vi "RSZVB Set Converter Source Frequency.vi"(4 "Numerator":i32, 5 "Sweep Type (0)":i32(ring) items=["Sweep", "CW/Fixed"], 6 "Offset":dbl format="%^.3e", 7 "Denominator":i32, 8 "error in (no error)":errorcluster {"code" format="%.0x"}, 9 "Port (1)":i32=1, 10 "Channel (1)":i32=1, 11 "VISA session":refnum<visa-resource-name>) -> (0 "error out":errorcluster {"code" format="%.0x"}, 3 "dup VISA session":refnum<visa-resource-name>)   [LabVIEW 2011]
doc: "Defines the converter source frequency at the converter port <Pt>.\n\nNotes:\n\n(1) This command is available for frequency converters with electronic attenuators R&S ZVA-ZxxxE.\n\nRemote-control command(s):\nSOURce<Ch>:FREQuency<Pt>:CONVersion:ARBitrary:CFRequency <numerator>, <denominator>, <offset>, CW | FIXed | SWEep"
uses:
  _utility/RSZVB Global Data.vi
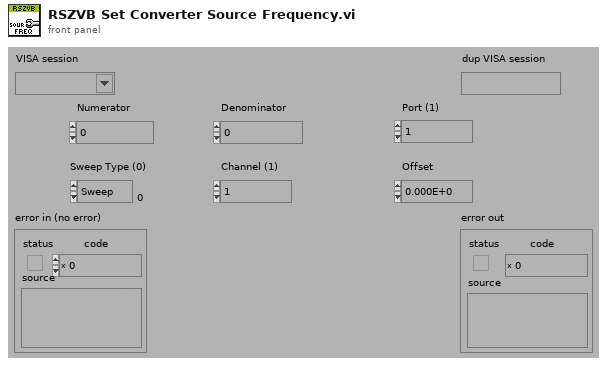
[diagram p1: front panel]
types:
  T1 = cluster{"Error Checking (T: On)":bool, "Installed Options":string[], "Data Valid?":bool, "Ports":i32, "Model":string[], "Option Checking (T: On)":bool}[]
  T2 = cluster{"Error Checking (T: On)":bool, "Installed Options":string[], "Data Valid?":bool, "Ports":i32, "Model":string[], "Option Checking (T: On)":bool}
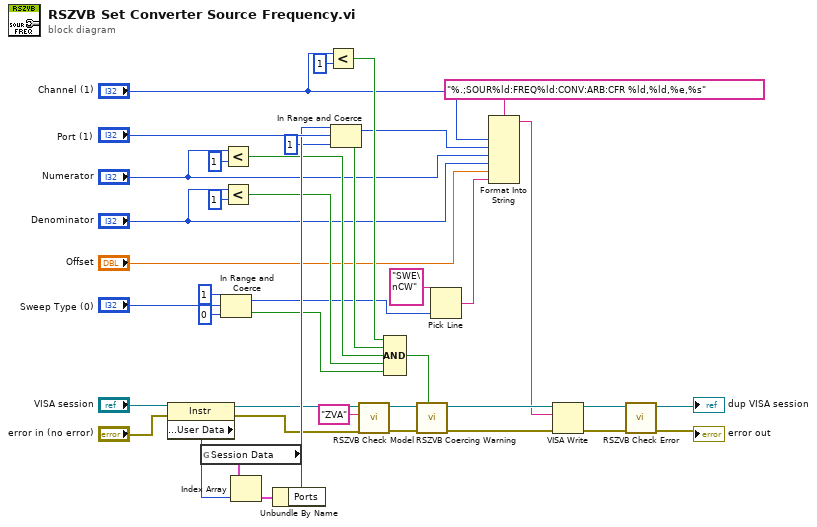
[diagram p0: block diagram]
diagram:
  n1 = property class="Instr"(reference="VISA session", error in="error in (no error)") -> (reference out=w4:refnum<visa-resource-name>, error out=w5:errorcluster, "General Settings:User Data"=w39:u32)
  n2 = global read "RSZVB Global Data.vi" "Session Data"() -> (w40:T1)
  n3 = In Range and Coerce(upper limit=1, x="Sweep Type (0)", lower limit=0) -> (coerced(x)=w14:i32, In Range?=w23:bool)
  n4 = Less?(x="Numerator", y=1) -> (x < y?=w25:bool)
  n5 = Less?(x="Denominator", y=1) -> (x < y?=w24:bool)
  n6 = Index Array(array=w40, index=w39) -> (element=w41:T2)
  n7 = Unbundle By Name(w41) -> ("Ports"=w35:i32)
  n8 = Less?(x="Channel (1)", y=1) -> (x < y?=w27:bool)
  n9 = In Range and Coerce(upper limit=w35, x="Port (1)", lower limit=1) -> (coerced(x)=w19:i32, In Range?=w26:bool)
  n10 = call "RSZVB Check Model.vi"("error in (no error)"=w5, "Model"="ZVA", "VISA session"=w4) -> ("error out"=w2:errorcluster, "dup VISA session"=w1:refnum<visa-resource-name>)  [unwired: 7 in]
  n11 = Compound Arithmetic op=AND(w27, w26, w25, w24, w23) -> (w22:bool)
  n12 = call "RSZVB Coercing Warning.vi"("In Range?"=w22, "error in (no error)"=w2, "VISA session"=w1) -> ("error out"=w12:errorcluster, "dup VISA session"=w11:refnum<visa-resource-name>)  [unwired: 7 in]
  n13 = Pick Line(multi-line string="SWE\nCW", line index=w14) -> (output string=w13:string)  [unwired: 1 in]
  n14 = Format Into String(format string="%.;SOUR%ld:FREQ%ld:CONV:ARB:CFR %ld,%ld,%e,%s", "Channel (1)", w19, "Numerator", "Denominator", "Offset", w13) -> (resulting string=w10:string)  [unwired: 2 in, 1 out]
  n15 = VISA Write(VISA resource name=w11, write buffer=w10, error in (no error)=w12) -> (VISA resource name out=w8:refnum<visa-resource-name>, error out=w9:errorcluster)  [unwired: 1 out]
  n16 = call "RSZVB Check Error.vi"("error in (no error)"=w9, "VISA session"=w8) -> ("error out"=→"error out":errorcluster, "dup VISA session"=→"dup VISA session":refnum<visa-resource-name>)  [unwired: 8 in]
